vi "temp_password.vi"() -> ()   [LabVIEW 2021]
panel:
  in  "Password":string
  in  "stop":bool
  out "Access Granted":bool
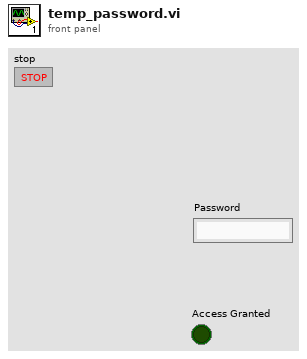
[diagram p1: front panel]
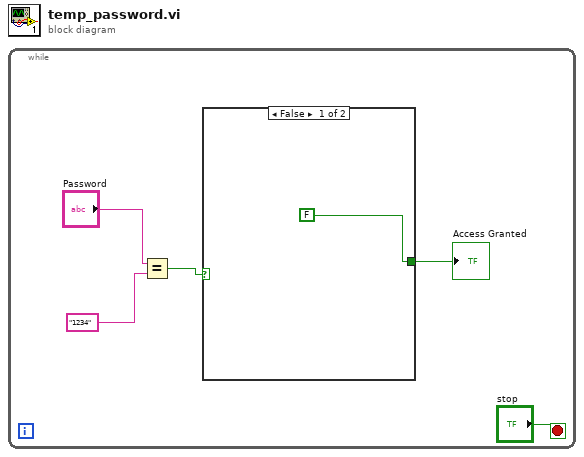
[diagram p0: block diagram]
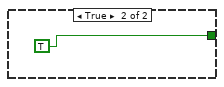
[diagram p2: hidden frame]
diagram:
  n1 = while {
    stop <- "stop" stop-if-true
    n2 = Equal?(x="Password", y="1234") -> (x = y?=w4:bool)
    n3 = case shown="False" w4 {
      tunnel: [FALSE TRUE] -> w3
      frame False {
      }
      frame True {
      }
    }
    "Access Granted" <- w3
  }
